vi "Ramp Up or Down With Delay.vi"(0 "Array":dbl[][](array[numeric]), 2 "Down at end":bool, 5 "Delay (ms)":dbl, 7 "Sampling rate (Hz)":dbl, 9 "Ramp (ms)":dbl=5.0, 11 "Ramp up?":bool=TRUE, 12 "Start (0)":dbl, 13 "End (1)":dbl=1.0) -> (4 "Ramped array":dbl[][](array[numeric]))   [LabVIEW 2020]
uses:
  PXI DAQ VIs/Utility VIs/Array Dimensions (2D).vi
  <vilib>/Analysis/NI_AALBase.lvlib
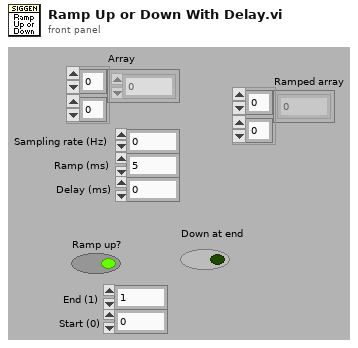
[diagram p1: front panel]
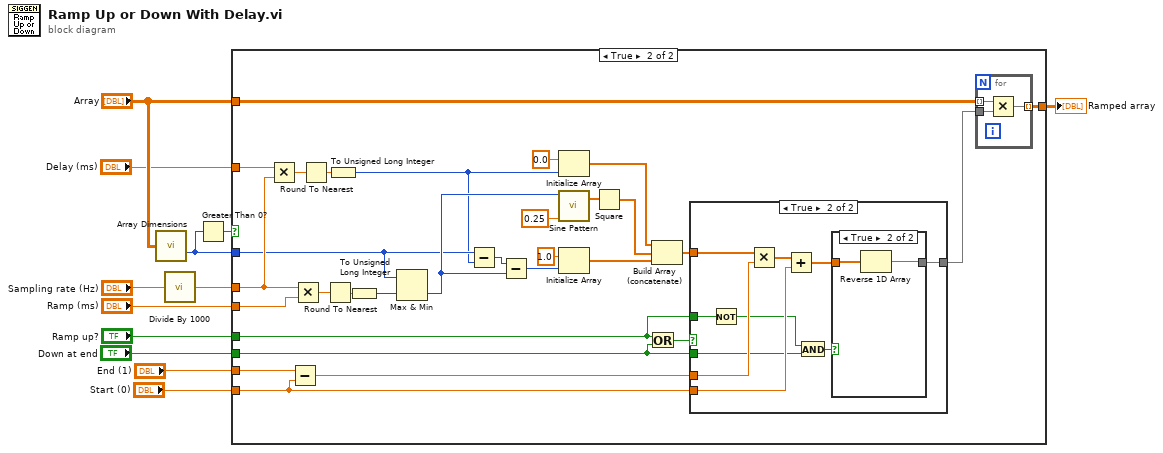
[diagram p0: block diagram]
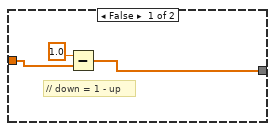
[diagram p3: hidden frame]
diagram:
  n1 = call-poly "Array Dimensions.vi"("2D Array"="Array") -> ("# columns"=w3:i32)  [unwired: 13 in, 1 out]
  n2 = call "Divide By 1000.vi"("X"="Sampling rate (Hz)") -> ("X/1000"=w2:dbl)
  n3 = Greater Than 0?(x=w3) -> (x > 0?=w9:bool)
  n4 = case shown="True" w9 {
    tunnel: "Ramp up?" -> [_ w14]
    tunnel: w2 -> [_ w22]
    tunnel: "Ramp (ms)" -> [_ w35]
    tunnel: w3 -> [_ w17]
    tunnel: "Array" -> [w13 w31]
    tunnel: [w13 w30] -> w7
    tunnel: "Start (0)" -> [_ w28]
    tunnel: "End (1)" -> [_ w29]
    tunnel: "Down at end" -> [_ w25]
    tunnel: "Delay (ms)" -> [_ w21]
    frame False {
    }
    frame True {
      n5 = Multiply(x=w21, y=w22) -> (x*y=w23:dbl)
      n6 = Subtract(x=w29, y=w28) -> (x-y=w27:dbl)
      n7 = Multiply(x=w22, y=w35) -> (x*y=w37:dbl)
      n8 = Round To Nearest(number=w23) -> (nearest integer value=w24:dbl)
      n9 = Round To Nearest(number=w37) -> (nearest integer value=w43:dbl)
      n10 = To Unsigned Long Integer(number=w24) -> (unsigned 32bit integer=w16:u32)
      n11 = To Unsigned Long Integer(number=w43) -> (unsigned 32bit integer=w32:u32)
      n12 = Max & Min(x=w17, y=w32) -> (min(x,y)=w42:u32)  [unwired: 1 out]
      n13 = Subtract(x=w17, y=w16) -> (x-y=w18:u32)
      n14 = Subtract(x=w18, y=w42) -> (x-y=w41:u32)
      n15 = Initialize Array(0.0 ("element"), w16) -> (w19:dbl[])
      n16 = call <vilib>:"Sine Pattern.vi"("cycles"=0.25, "samples"=w42) -> ("Sinusoidal Pattern"=w34:dbl[])  [unwired: 2 in, 1 out]
      n17 = Initialize Array(1.0 ("element"), w41) -> (w39:dbl[])
      n18 = Square(x=w34) -> (x^2=w33:dbl[])
      n19 = Or(x=w14, y=w25) -> (x .or. y?=w26:bool)
      n20 = Build Array (concatenate)(w19, w33, w39) -> (w38:dbl[])
      n21 = case shown="True" w26 {
        tunnel: w38 -> [w45 w56]
        tunnel: [w44 w51] -> w15
        tunnel: w28 -> [_ w55]
        tunnel: w27 -> [_ w53]
        tunnel: w25 -> [_ w50]
        tunnel: w14 -> [_ w48]
        frame False {
          # "// down = 1 - up"
          n22 = Subtract(x=1.0, y=w45) -> (x-y=w44:dbl[])
        }
        frame True {
          n23 = Not(x=w48) -> (.not. x?=w47:bool)
          n24 = Multiply(x=w56, y=w53) -> (x*y=w54:dbl[])
          n25 = Add(x=w54, y=w55) -> (x+y=w52:dbl[])
          n26 = And(x=w47, y=w50) -> (x .and. y?=w49:bool)
          n27 = case shown="True" w49 {
            tunnel: w52 -> [w57 w59]
            tunnel: [w57 w58] -> w51
            frame False {
            }
            frame True {
              n28 = Reverse 1D Array(array=w59) -> (reversed array=w58:dbl[])
            }
          }
        }
      }
      n29 = for {
        tunnel: w31 -> [w62] mode=indexing
        tunnel: w15 -> [w61]
        tunnel: [w60] -> w30 mode=indexing
        n30 = Multiply(x=w62, y=w61) -> (x*y=w60:dbl[])
      }
    }
  }
  "Ramped array" <- w7
